vi "Get Server Stop UE.vi"(11 "OOP Server in":refnum<class "Template Server.lvclass">) -> (2 "Server Stop UE":refnum<user-event>, 3 "OOP Server out":refnum<class "Template Server.lvclass">)   [LabVIEW 2019, in "Template Server.lvlib" / "Template Server.lvclass"]
uses:
  Template Server.lvclass
  Template Server.lvclass/Template Server.ctl
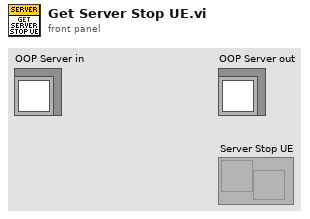
[diagram p1: front panel]
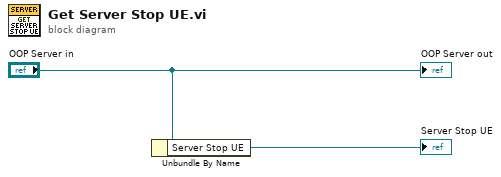
[diagram p0: block diagram]
diagram:
  n1 = Unbundle By Name("OOP Server in") -> ("Server Stop UE"=→"Server Stop UE":refnum<user-event>)
  "OOP Server out" <- "OOP Server in"
